vi "Run Action.vi"(7 "Logger":refnum<class "Logger.lvclass">, 8 "error in (no error)":errorcluster, 10 "Package":refnum<class "PackageAbstract.lvclass">, 11 "UpdateAction in":refnum<class "DependAction.lvclass">) -> (0 "error out":errorcluster, 2 "Problems":string[](array[string]), 3 "UpdateAction out":refnum<class "DependAction.lvclass">)   [LabVIEW 2020, in "GPackTools.lvlib" / "DependAction.lvclass"]
uses:
  DependAction.lvclass
  GPack/PackageAbstract/PackageAbstract.lvclass
  GPack/Logger/Logger.lvclass
  DependAction.lvclass/DependAction.ctl
  GPack/NamedPackage/NamedPackage.lvclass
  <vilib>/regexp/Match Regular Expression.xnode
  GPackTools.lvlib
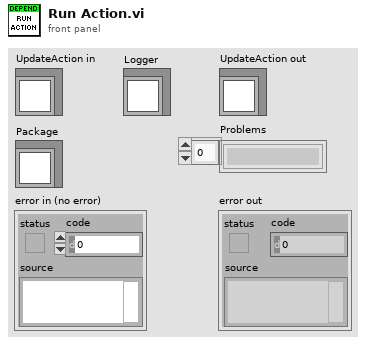
[diagram p1: front panel]
types:
  T1 = typedef "GPack.lvlib/Dependency.ctl" = cluster{"Info":T2, "Path":path}
  T2 = typedef "GPack.lvlib/Package Info.ctl" = cluster{"Name":string, "Type":string, "Host":string, "Path":string, "Branch":string, "Version":string, "License":string}
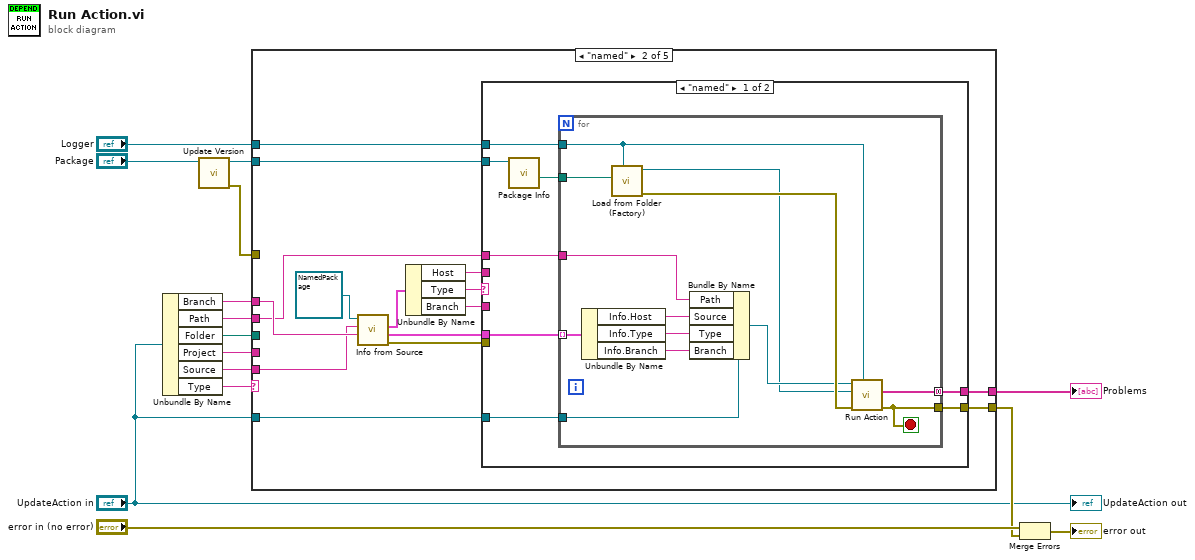
[diagram p0: block diagram]
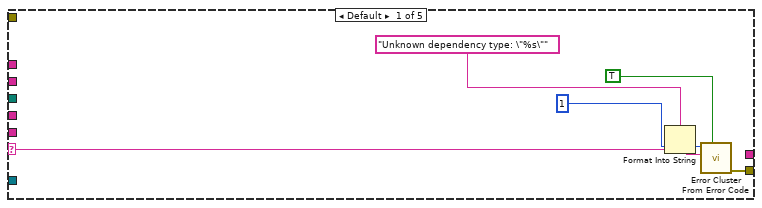
[diagram p2: hidden frame]
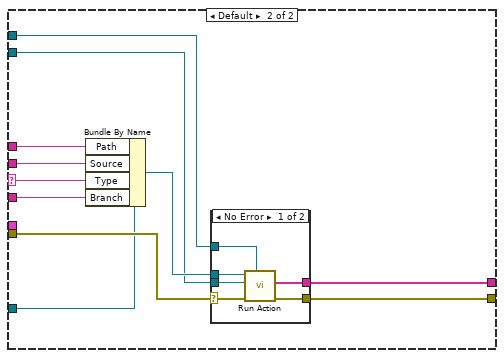
[diagram p3: hidden frame]
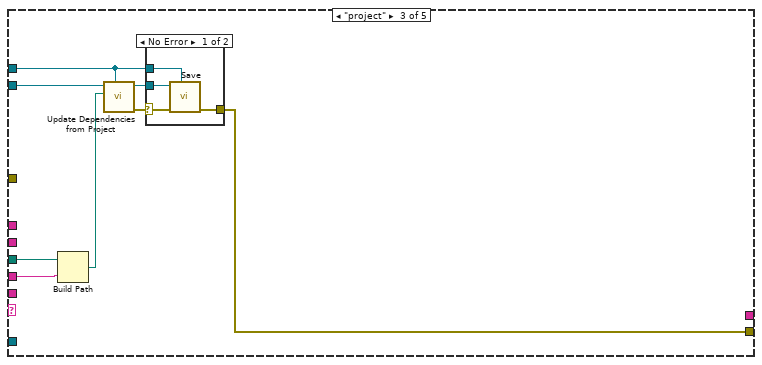
[diagram p5: hidden frame]
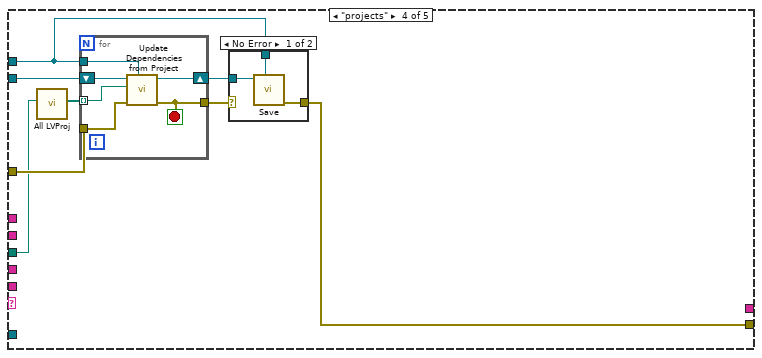
[diagram p7: hidden frame]
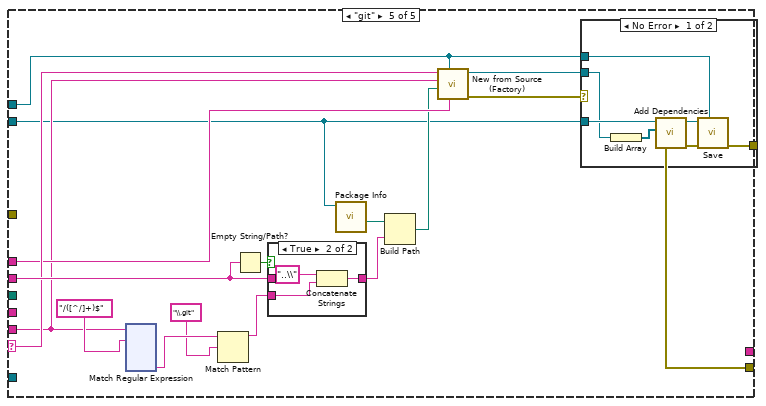
[diagram p9: hidden frame]
diagram:
  n1 = Unbundle By Name("UpdateAction in") -> ("Branch"=w4:string, "Path"=w5:string, "Folder"=w9:path, "Project"=w12:string, "Source"=w13:string, "Type"=w14:string)
  n2 = call-dynamic "Update Version.vi"("Package in"="Package") -> ("error out"=w6:errorcluster, "Package out"=w7:refnum<class "PackageAbstract.lvclass">)  [unwired: 9 in]
  n3 = case shown="\"named\"" w14 {
    selector: w14 -> [w17 _ _ _ w120]
    tunnel: w13 -> [_ w30 _ _ w113]
    tunnel: w12 -> [_ _ w83 _ _]
    tunnel: w7 -> [_ w24 w81 w94 w111]
    tunnel: w9 -> [_ _ w82 w95 _]
    tunnel: "Logger" -> [_ w25 w79 w89 w107]
    tunnel: w6 -> [_ _ _ w96 _]
    tunnel: w5 -> [_ w29 _ _ w122]
    tunnel: w4 -> [_ w31 _ _ w114]
    tunnel: [w21 w27 w80 w90 w109] -> w3
    tunnel: "UpdateAction in" -> [_ w26 _ _ _]
    tunnel: [_ w23 _ _ _] -> w1
    frame Default {
      n4 = Format Into String(format string="Unknown dependency type: \"%s\"", w17) -> (resulting string=w16:string)  [unwired: 2 in, 1 out]
      n5 = call <vilib>:"Error Cluster From Error Code.vi"("show call chain? (False)"=TRUE, "error message (\"\")"=w16, "error code (0)"=1) -> ("error out"=w21:errorcluster)  [unwired: 6 in]
    }
    frame "named" {
      n6 = call-dynamic "Info from Source.vi"("Branch (Default)"=w31, "Source"=w30, "NamedPackage in"=refnum<class "NamedPackage.lvclass"> refnum) -> ("error out"=w28:errorcluster, "Dependencies"=w22:T1[], "Package Info"=w35:T2)  [unwired: 5 in, 1 out]
      n7 = Unbundle By Name(w35) -> ("Host"=w34:string, "Type"=w33:string, "Branch"=w32:string)
      n8 = case shown="\"named\"" w33 {
        selector: w33 -> [_ w67]
        tunnel: w34 -> [_ w68]
        tunnel: w32 -> [_ w66]
        tunnel: w29 -> [w39 w65]
        tunnel: w28 -> [_ w64]
        tunnel: [w40 w63] -> w27
        tunnel: w26 -> [w43 w62]
        tunnel: w25 -> [w42 w60]
        tunnel: w24 -> [w38 w59]
        tunnel: [w41 w58] -> w23
        tunnel: w22 -> [w44 _]
        frame "named" {
          n9 = call-dynamic "Package Info.vi"("Package in"=w38) -> ("Folder"=w37:path)  [unwired: 8 in, 2 out]
          n10 = for {
            tunnel: w44 -> [w54] mode=indexing
            tunnel: w43 -> [w49]
            tunnel: w42 -> [w46]
            tunnel: [w56] -> w41 mode=concatenating
            tunnel: [w55] -> w40
            tunnel: w39 -> [w53]
            tunnel: w37 -> [w47]
            stop <- w55 stop-if-true
            n11 = Unbundle By Name(w54) -> ("Info.Host"=w52:string, "Info.Type"=w51:string, "Info.Branch"=w50:string)
            n12 = call "Load from Folder (Factory).vi"("Logger"=w46, "Folder"=w47) -> ("error out"=w57:errorcluster, "PackageAbstract out"=w45:refnum<class "PackageAbstract.lvclass">)  [unwired: 8 in]
            n13 = Bundle By Name(cluster=w49, "Path"=w53, "Source"=w52, "Type"=w51, "Branch"=w50) -> (w48:refnum<class "DependAction.lvclass">)
            n14 = call-dynamic "Run Action.vi"("Logger"=w46, "error in (no error)"=w57, "Package"=w45, "UpdateAction in"=w48) -> ("error out"=w55:errorcluster, "Problems"=w56:string[])  [unwired: 5 in, 1 out]
          }
        }
        frame Default {
          n15 = Bundle By Name(cluster=w62, "Path"=w65, "Source"=w68, "Type"=w67, "Branch"=w66) -> (w61:refnum<class "DependAction.lvclass">)
          n16 = case shown="No Error" w64 {
            selector: w64 -> [w74 w75]
            tunnel: [w73 w75] -> w63
            tunnel: w61 -> [w72 _]
            tunnel: w60 -> [w71 _]
            tunnel: w59 -> [w70 _]
            tunnel: [w69 _] -> w58
            frame No Error {
              n17 = call-dynamic "Run Action.vi"("Logger"=w71, "error in (no error)"=w74, "Package"=w70, "UpdateAction in"=w72) -> ("error out"=w73:errorcluster, "Problems"=w69:string[])  [unwired: 5 in, 1 out]
            }
            frame Error {
            }
          }
        }
      }
    }
    frame "project" {
      n18 = Build Path(base path=w82, name or relative path=w83) -> (appended path=w78:path)
      n19 = call "Update Dependencies from Project.vi"("Logger"=w79, "lvproj Path"=w78, "PackageAbstract in"=w81) -> ("error out"=w77:errorcluster, "PackageAbstract out"=w76:refnum<class "PackageAbstract.lvclass">)  [unwired: 7 in]
      n20 = case shown="No Error" w77 {
        selector: w77 -> [w86 w88]
        tunnel: w76 -> [w87 _]
        tunnel: [w85 w88] -> w80
        tunnel: w79 -> [w84 _]
        frame No Error {
          n21 = call "Save.vi"("Logger"=w84, "error in (no error)"=w86, "PackageAbstract in"=w87) -> ("error out"=w85:errorcluster)  [unwired: 7 in, 1 out]
        }
        frame Error {
        }
      }
    }
    frame "projects" {
      n22 = call "All LVProj.vi"("Folder"=w95) -> ("All LVProj"=w93:path[])  [unwired: 10 in]
      n23 = for {
        shift-right: [w105] -> w91
        shift-left: w94 -> [w106]
        tunnel: w93 -> [w104] mode=indexing
        tunnel: [w103] -> w92
        tunnel: w89 -> [w102]
        tunnel: w96 -> [w101]
        stop <- w103 stop-if-true
        n24 = call "Update Dependencies from Project.vi"("Logger"=w102, "error in (no error)"=w101, "lvproj Path"=w104, "PackageAbstract in"=w106) -> ("error out"=w103:errorcluster, "PackageAbstract out"=w105:refnum<class "PackageAbstract.lvclass">)  [unwired: 6 in]
      }
      n25 = case shown="No Error" w92 {
        selector: w92 -> [_ w100]
        tunnel: w91 -> [w99 _]
        tunnel: [w98 w100] -> w90
        tunnel: w89 -> [w97 _]
        frame No Error {
          n26 = call "Save.vi"("Logger"=w97, "PackageAbstract in"=w99) -> ("error out"=w98:errorcluster)  [unwired: 8 in, 1 out]
        }
        frame Error {
        }
      }
    }
    frame "git" {
      n27 = xnode "Match Regular Expression"("input string"=w113, "regular expression"="/([^/]+)$") -> ("submatch 1"=w118:string)  [unwired: 4 in, 5 out]
      n28 = Match Pattern(string=w118, regular expression="\\.git") -> (before substring=w121:string)  [unwired: 1 in, 3 out]
      n29 = Empty String/Path?(string/path=w122) -> (empty?=w123:bool)
      n30 = case shown="True" w123 {
        tunnel: w121 -> [_ w250]
        tunnel: w122 -> [w248 _]
        tunnel: [w248 w249] -> w115
        frame False {
        }
        frame True {
          n31 = Concatenate Strings("..\\" ("string"), w250) -> (w249:string)
        }
      }
      n32 = call-dynamic "Package Info.vi"("Package in"=w111) -> ("Folder"=w116:path)  [unwired: 8 in, 2 out]
      n33 = Build Path(base path=w116, name or relative path=w115) -> (appended path=w112:path)
      n34 = call "New from Source (Factory).vi"("Branch (Default)"=w114, "Logger"=w107, "Folder"=w112, "Source"=w113, "Type"=w120) -> ("error out"=w108:errorcluster, "PackageAbstract out"=w110:refnum<class "PackageAbstract.lvclass">)  [unwired: 5 in]
      n35 = case shown="No Error" w108 {
        selector: w108 -> [_ w131]
        tunnel: w111 -> [w127 _]
        tunnel: w110 -> [w126 _]
        tunnel: [w125 w131] -> w109
        tunnel: w107 -> [w124 _]
        frame No Error {
          n36 = Build Array(w126) -> (w130:refnum<class "PackageAbstract.lvclass">[])
          n37 = call "Add Dependencies.vi"("Dependencies"=w130, "PackageAbstract in"=w127) -> ("error out"=w128:errorcluster, "PackageAbstract out"=w129:refnum<class "PackageAbstract.lvclass">)  [unwired: 8 in]
          n38 = call "Save.vi"("Logger"=w124, "error in (no error)"=w128, "PackageAbstract in"=w129) -> ("error out"=w125:errorcluster)  [unwired: 7 in, 1 out]
        }
        frame Error {
        }
      }
    }
  }
  "Problems" <- w1
  n39 = Merge Errors("error in (no error)", w3) -> (→"error out":errorcluster)
  "UpdateAction out" <- "UpdateAction in"
